vi "Init_Robot(SubVI).vi"(11 "IP address":string) -> (0 "error out":errorcluster, 2 "Current_Position":T1, 3 "FPGA starter kit host 2.0 out":refnum<class "NI_Robotics_Starter Kit Host_9632_2.0.lvclass">)   [LabVIEW 2017]
uses:
  Ctl/Current_Position.ctl
  <vilib>/robotics/Starter Kit/2.0/9632 Host Interface/NI_Robotics_Starter Kit Host_9632_2.0.lvclass
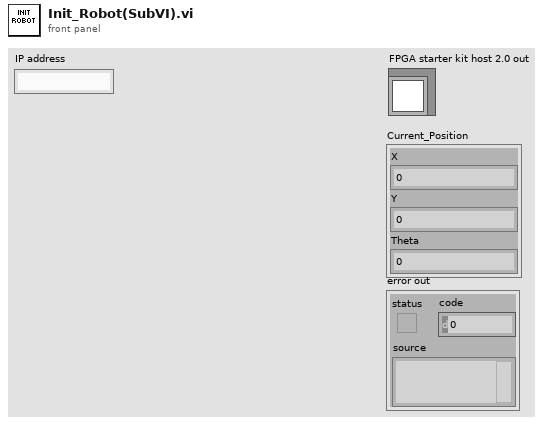
[diagram p1: front panel]
types:
  T1 = typedef "Current_Position.ctl" = cluster{"X":dbl, "Y":dbl, "Theta":dbl}
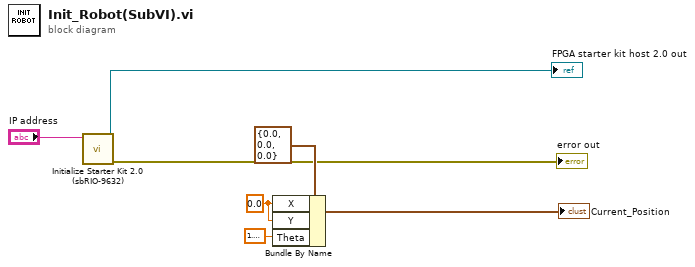
[diagram p0: block diagram]
diagram:
  w2 = 0.0 ("X")
  n1 = call <vilib>:"Initialize Starter Kit 2.0 (sbRIO-9632).vi"("IP address (\"\")"="IP address") -> ("error out"=→"error out":errorcluster, "FPGA starter kit host 2.0 out"=→"FPGA starter kit host 2.0 out":refnum<class "NI_Robotics_Starter Kit Host_9632_2.0.lvclass">)  [unwired: 9 in]
  n2 = Bundle By Name(cluster=T1 {"X"=0.0, "Y"=0.0, "Theta"=0.0} ("Current_Position"), "X"=w2, "Y"=w2, "Theta"=1.5707963267948966) -> (→"Current_Position":T1)
